vi "MoveTW.vi"(8 "error in (no error)":errorcluster, 10 "Angle":dbl) -> (0 "error out":errorcluster)   [LabVIEW 2015]
uses:
  TW Global.vi
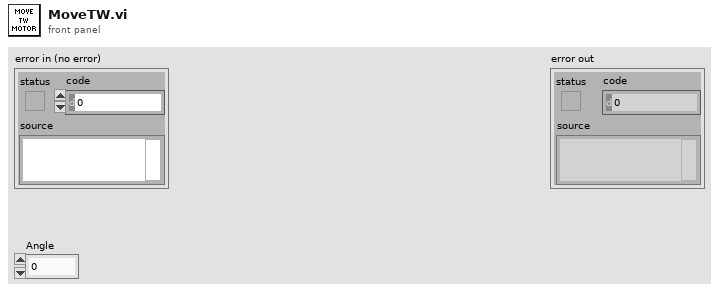
[diagram p1: front panel]
types:
  T1 = typedef "Detailed Motor Type Def.ctl" = cluster{"MotorRef":T2, "Encoder Ticks Per Rev":dbl, "Set Position":dbl, "Wheel Radius":dbl}
  T2 = typedef "WPI_MotorControlDeviceRef.ctl" = cluster{"DeviceStatus":errorcluster, "Type":T3, "PWM":cluster{"PWM Channel":T4, "DeadBand":T5}, "CAN":cluster{"Device Number":u8, "Control Mode":T6, "Semaphore":T7, "Max Vout":dbl, "TalonSRX Control Mode":T8}, "Invert":bool}
  T3 = typedef "WPI_MotorControlType.ctl" = enum16{"PWM", "CAN", "CANTalonSRX"}
  T4 = typedef "FPGA_DIOPWMChannel.ctl" = enum8{"PWM 0", "PWM 1", "PWM 2", "PWM 3", "PWM 4", "PWM 5", "PWM 6", "PWM 7", "PWM 8", "PWM 9", "PWM MXP 0", "PWM MXP 1", "PWM MXP 2", "PWM MXP 3", "PWM MXP 4", "PWM MXP 5", "PWM MXP 6", "PWM MXP 7", "PWM MXP 8", "PWM MXP 9", "Invalid"}
  T5 = typedef "WPI_PWMDeadband.ctl" = cluster{"Name":string, "maxPositivePwm":i32, "minPositivePwm":i32, "centerPwm":i32, "maxNegativePwm":i32, "minNegativePwm":i32, "angularRange":u16}
  T6 = typedef "WPI_CANJaguar_ControlMode.ctl" = enum8{"Percent VBus", "Current", "Speed", "Position", "Voltage"}
  T7 = typedef "Semaphore RefNum" = refnum<k1>
  T8 = typedef "WPI_CANTalonSRX_APIControlMode.ctl" = enum8{"Percent VBus", "Speed", "Position", "Slave", "Unchanged / Invalid", "Voltage Compensation", "Current", "Motion Profile"}
  T9 = typedef "PortC Settings Type Def.ctl" = cluster{"Down":dbl, "Up":dbl, "Increments":dbl}
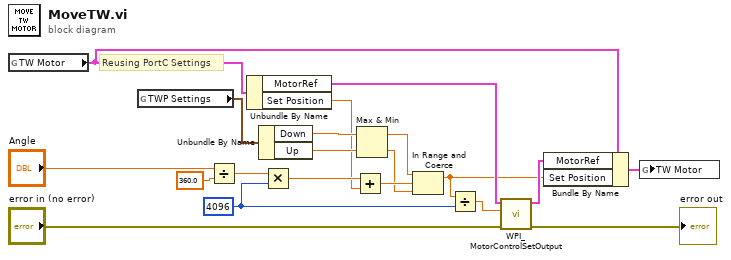
[diagram p0: block diagram]
diagram:
  w4 = 4096
  # "Reusing PortC Settings"
  n1 = global read "TW Global.vi" "TW Motor"() -> (w1:T1)
  n2 = global read "TW Global.vi" "TWP Settings"() -> (w11:T9)
  n3 = Divide(x="Angle", y=360.0) -> (x/y=w10:dbl)
  n4 = Unbundle By Name(w1) -> ("MotorRef"=w19:T2, "Set Position"=w3:dbl)
  n5 = Unbundle By Name(w11) -> ("Down"=w13:dbl, "Up"=w12:dbl)
  n6 = Multiply(x=w10, y=w4) -> (x*y=w5:dbl)
  n7 = Add(x=w5, y=w3) -> (x+y=w15:dbl)
  n8 = Max & Min(x=w13, y=w12) -> (max(x,y)=w6:dbl, min(x,y)=w7:dbl)
  n9 = In Range and Coerce(upper limit=w6, x=w15, lower limit=w7) -> (coerced(x)=w14:dbl)  [unwired: 1 out]
  n10 = Divide(x=w14, y=w4) -> (x/y=w20:dbl)
  n11 = call <vilib>:"WPI_MotorControlSetOutput.vi"("error in (no error)"="error in (no error)", "Output"=w20, "MotorControlDevRef"=w19) -> ("error out"=→"error out":errorcluster, "MotorControlDevRef"=w16:T2)  [unwired: 6 in, 1 out]
  n12 = Bundle By Name(cluster=w1, "MotorRef"=w16, "Set Position"=w14) -> (w2:T1)
  n13 = global write "TW Global.vi" "TW Motor"(w2) -> ()
